vi "Timer FGV.vi"(8 "Error In":errorcluster, 10 "Time Target":dbl format="%#_13g", 11 "State":enum16{"Reset", "Read", "Pause"}(ring)=enum."Pause") -> (0 "Error Out":errorcluster, 2 "Time Elapsed":bool, 3 "Elapsed Time":dbl)   [LabVIEW 2016]
doc: "This is the timer VI to calculate elapsed time and pause time."
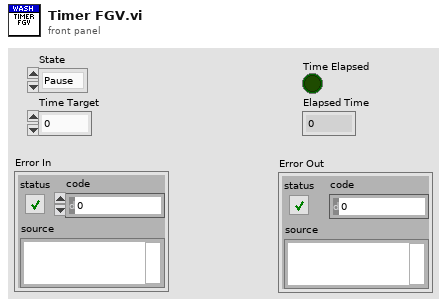
[diagram p1: front panel]
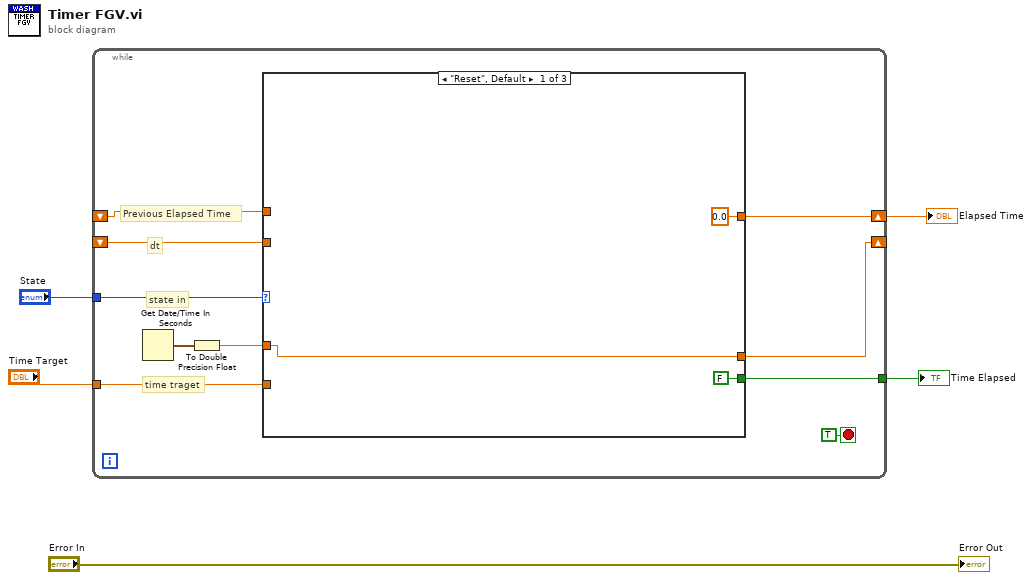
[diagram p0: block diagram]
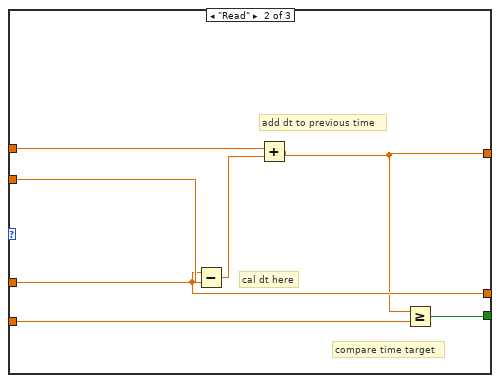
[diagram p2: hidden frame]
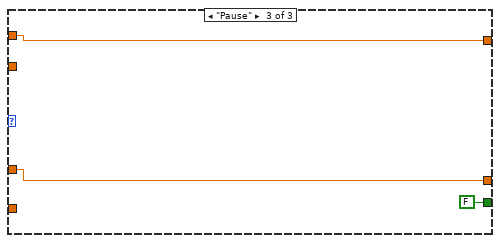
[diagram p3: hidden frame]
diagram:
  n1 = while {
    tunnel: "State" -> [w15]
    shift-right: [w9] -> _
    shift-left: _ -> [w11]
    tunnel: "Time Target" -> [w8]
    tunnel: [w7] -> w3
    shift-right: [w10] -> w2
    shift-left: _ -> [w6]
    stop <- TRUE stop-if-true
    # "time traget"
    # "state in"
    # "dt"
    # "Previous Elapsed Time"
    n2 = Get Date/Time In Seconds() -> (seconds since 1Jan1904=w13:timestamp)
    n3 = To Double Precision Float(number=w13) -> (double precision float=w12:dbl)
    n4 = case shown="\"Reset\", Default" w15 {
      tunnel: w12 -> [w16 w22 w27]
      tunnel: w11 -> [_ w25 _]
      tunnel: w6 -> [_ w23 w28]
      tunnel: [0.0 w21 w28] -> w10
      tunnel: [w16 w22 w27] -> w9
      tunnel: w8 -> [_ w20 _]
      tunnel: [FALSE w19 FALSE] -> w7
      frame "Reset", Default {
      }
      frame "Read" {
        # "compare time target"
        # "add dt to previous time"
        # "cal dt here"
        n5 = Subtract(x=w22, y=w25) -> (x-y=w24:dbl)
        n6 = Add(x=w23, y=w24) -> (x+y=w21:dbl)
        n7 = Greater Or Equal?(x=w21, y=w20) -> (x >= y?=w19:bool)
      }
      frame "Pause" {
      }
    }
  }
  "Time Elapsed" <- w3
  "Elapsed Time" <- w2
  "Error Out" <- "Error In"
